vi "FTW-Inbox-Construct.vi"(5 "Primary Inbox Address":string, 7 "Inbox Configuration":string, 11 "error in":errorcluster) -> (4 "FTW Actor Inbox":T1, 6 "Resolved Primary Inbox Address":string, 8 "Incoming Request":refnum<event-registration>, 15 "error out":errorcluster)   [LabVIEW 2015]
uses:
  core/type/FTW-Type-Actor-Inbox.ctl
  json/core/FTW-JSON-Core-Structure.ctl
panel:
  in  "Statistics":refnum<data-value>
  in  "Actor Identity":string
  # "Inputs"
  # "Outputs"
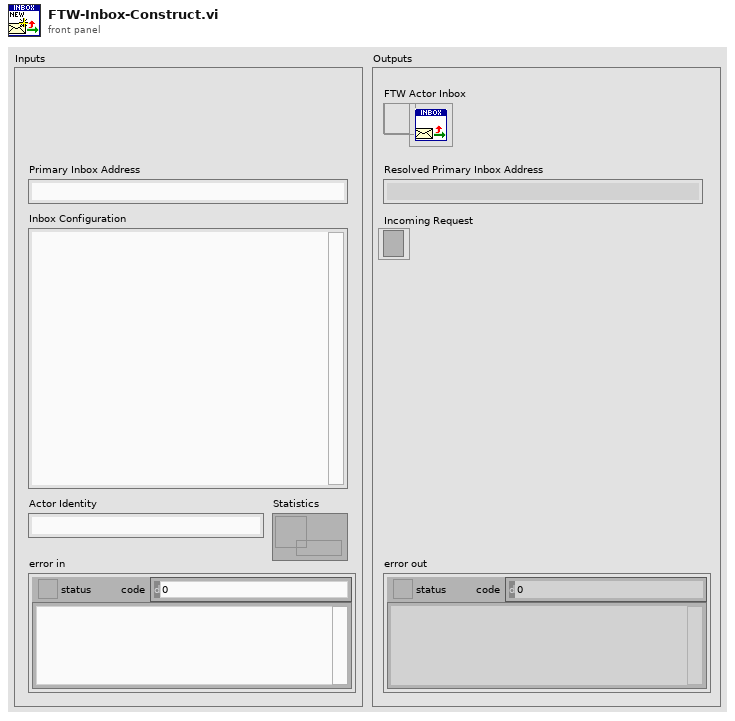
[diagram p1: front panel]
types:
  T1 = typedef "FTW-Type-Actor-Inbox.ctl" = refnum<data-value>
  T2 = typedef "FTW-Inbox-Core-RoutingRule.ctl" = cluster{"Pattern":string, "BusyTimeout":i32, "SendTimeout":i32, "Accept":bool, "Reject":bool, "ReplyWithIdentity":bool, "ReplyWithStats":bool, "ReplyWithTimestamp":bool, "ReplyWithRelativeTimer":bool, "AutoReply":bool}
  T3 = cluster{"FTW-CodeGen-Type":enum16{"FTW-Actor-Inbox"}, "Socket":i64}
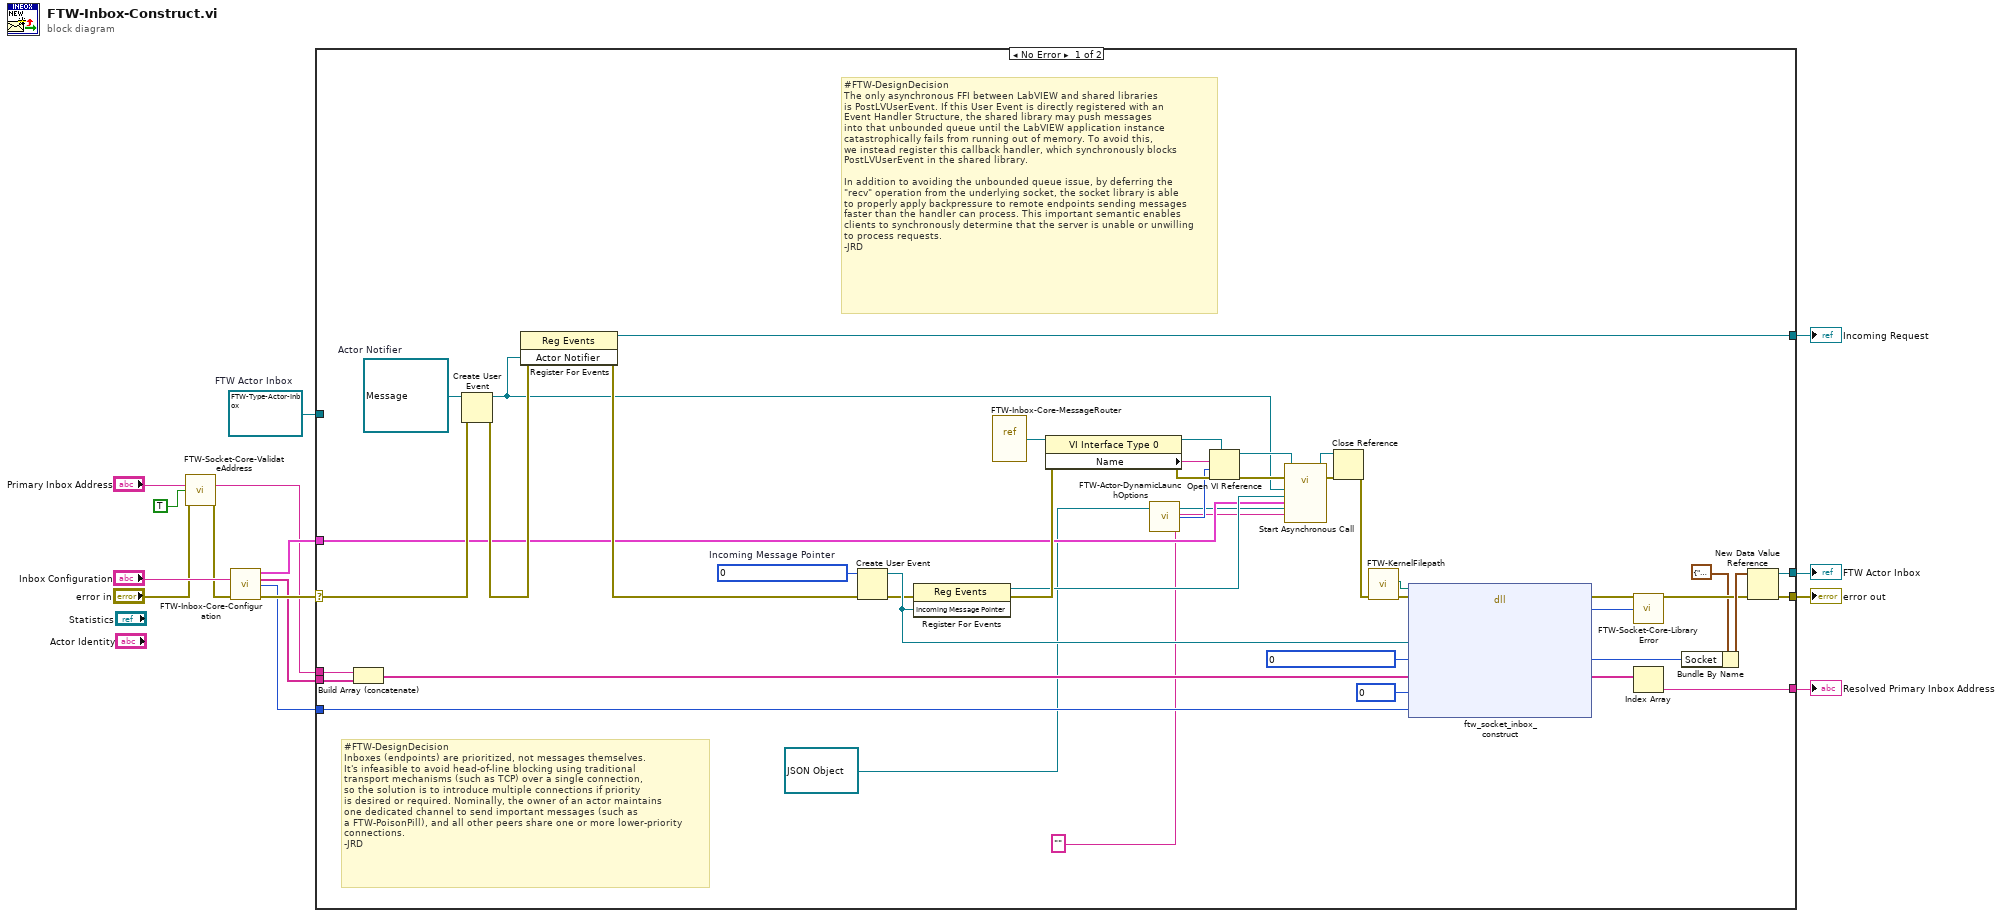
[diagram p0: block diagram]
diagram:
  w1 = T1 refnum  # FTW Actor Inbox
  n1 = call "FTW-Socket-Core-ValidateAddress.vi"("Address"="Primary Inbox Address", "Allow wildcard replacement?"=TRUE, "error in"="error in") -> ("Sanitized Address"=w5:string, "error out"=w6:errorcluster)  [unwired: 10 in, 1 out]
  n2 = call "FTW-Inbox-Core-Configuration.vi"("Inbox Configuration"="Inbox Configuration", "error in"=w6) -> ("Message Routing Rules"=w10:T2[], "Additional Endpoint Addresses"=w4:string[], "Receive Message Size Limit"=w3:i32, "error out"=w12:errorcluster)  [unwired: 9 in, 1 out]
  n3 = case shown="No Error" w12 {
    selector: w12 -> [w54 w59]
    tunnel: [w49 w58] -> w2
    tunnel: [w48 w59] -> w15
    tunnel: [w55 _] -> w13
    tunnel: w5 -> [w44 _]
    tunnel: [w40 _] -> w14
    tunnel: w3 -> [w46 _]
    tunnel: w10 -> [w20 _]
    tunnel: w4 -> [w42 _]
    tunnel: w1 -> [_ w58]
    frame No Error {
      w39 = i64 0  # Incoming Message Pointer
      w47 = refnum<queue> refnum  # Actor Notifier
      # "#FTW-DesignDecision\nThe only asynchronous FFI between LabVIEW and shared libraries\nis PostLVUserEvent. If this User Event is directly registered with an\nEvent Handler Structure, the shared library may push messages\ninto that unbounded queue until the LabVIEW application instance\ncatastrophically fails from running out of memory. To avoid this,\nwe instead register this callback handler, which synchronously blocks\nPostLVUserEvent in the shared library.\n\nIn addition to avoiding the unbounded queue issue, by deferring the\n\"recv\" operation from the underlying socket, the socket library is able\nto properly apply backpressure to remote endpoints sending messages\nfaster than the handler can process. This important semantic enables\nclients to synchronously determine that the server is unable or unwilling\nto process requests.\n-JRD"
      # "#FTW-DesignDecision\nInboxes (endpoints) are prioritized, not messages themselves.\nIt's infeasible to avoid head-of-line blocking using traditional\ntransport mechanisms (such as TCP) over a single connection,\nso the solution is to introduce multiple connections if priority\nis desired or required. Nominally, the owner of an actor maintains\none dedicated channel to send important messages (such as\na FTW-PoisonPill), and all other peers share one or more lower-priority\nconnections.\n-JRD"
      n4 = Build Array (concatenate)(w44, w42) -> (w43:string[])
      n5 = Create User Event(user event datatype=w47, error in=w54) -> (user event=w19:refnum<user-event>, error out=w53:errorcluster)
      n6 = register-events(error in=w53, w19) -> (reference out=w55:refnum<event-registration>, error out=w52:errorcluster)  [unwired: 1 in]
      n7 = Create User Event(user event datatype=w39, error in=w52) -> (user event=w25:refnum<user-event>, error out=w22:errorcluster)
      n8 = register-events(error in=w22, w25) -> (reference out=w21:refnum<event-registration>, error out=w26:errorcluster)  [unwired: 1 in]
      n9 = vi-ref "FTW-Inbox-Core-MessageRouter.vi"() -> (w36:refnum<vi>)
      n10 = property class="VI Interface Type 0"(reference=w36, error in=w26) -> (reference out=w34:refnum<vi>, error out=w28:errorcluster, "Name"=w35:string)
      n11 = call "FTW-Actor-DynamicLaunchOptions.vi"() -> ("Open VI Ref Options"=w27:i32)  [unwired: 1 in]
      n12 = Open VI Reference(type specifier VI Refnum (for type only)=w34, vi path=w35, options=w27, error in (no error)=w28) -> (vi reference=w33:refnum<vi>, error out=w30:errorcluster)  [unwired: 2 in]
      n13 = call-by-ref "Start Asynchronous Call"(reference=w33, error in=w30, "ActorNotifier"=w19, "Messages from Inbox Thread"=w21, "Routing Rules"=w20, "Statistics"=refnum<data-value> refnum, "Actor Identity"="") -> (reference out=w29:refnum<vi>, error out=w32:errorcluster)  [unwired: 11 in]
      n14 = Close Reference(reference=w29, error in (no error)=w32) -> (error out=w31:errorcluster)
      n15 = call "FTW-KernelFilepath.vi"("error in"=w31) -> ("error out"=w38:errorcluster, "Library Filepath"=w37:path)  [unwired: 8 in, 1 out]
      n16 = dll-call lib="?" fn="ftw_socket_inbox_construct"(path in=w37, error in=w38, "Incoming Message Broker"=w25, "Socket Handle"=i64 0, "Addresses"=w43, "Linger (msec)"=0, "Max Recv Size (bytes)"=w46) -> (error out=w57:errorcluster, "Return Value"=w56:i64, "Socket Handle"=w51:i64, "Addresses"=w41:string[])  [unwired: 6 in, 1 out]
      n17 = call "FTW-Socket-Core-LibraryError.vi"("error in"=w57, "Return Value"=w56) -> ("error out"=w23:errorcluster)  [unwired: 13 in]
      n18 = Index Array(array=w41) -> (element=w40:string)  [unwired: 1 in]
      n19 = Bundle By Name(cluster=T3 {"FTW-CodeGen-Type"=enum."FTW-Actor-Inbox", "Socket"=0}, "Socket"=w51) -> (w50:T3)
      n20 = New Data Value Reference(data value=w50, error in=w23) -> (data value reference=w49:refnum<data-value>, error out=w48:errorcluster)
    }
    frame Error {
    }
  }
  "error out" <- w15
  "FTW Actor Inbox" <- w2
  "Resolved Primary Inbox Address" <- w14
  "Incoming Request" <- w13
